vi "Update_Readback.vi"(8 "error in (no error)":errorcluster, 9 "Value":u32, 10 "PV URL":string, 11 "CS++IEFWerner in":refnum<class "CS++IEFWerner.lvclass">) -> (0 "error out":errorcluster, 3 "CS++IEFWerner out":refnum<class "CS++IEFWerner.lvclass">)   [LabVIEW 2015, in "CS++IEFWerner.lvlib" / "CS++IEFWerner.lvclass"]
doc: "This VI gets the infos from the Status SV of the IEF motor controller, makes some calculations and updates the important SVs."
uses:
  CS++IEFWerner.lvclass
  CS++IEFWerner.lvclass/CS++IEFWerner.ctl
  CSPP_Core/Classes/CS++ProcessVariables/ProcessVariable/PV.lvclass
  CSPP_Core/Classes/CS++ProcessVariables/ProcessVariable/PV.lvclass/PV.ctl
  CSPP_Core/Classes/CS++ProcessVariables/ProcessVariable/Write Data.vi
  CSPP_Core/Classes/CS++ProcessVariables/ProcessVariable/Write Timestamp.vi
  CSPP_Core/Classes/CS++ProcessVariables/PVConnection/PVConnection.lvclass
  CSPP_DeviceBase/CS++Motor/CS++Motor.lvclass
  instr.lib/IEF-pac/IEF Werner.lvlib
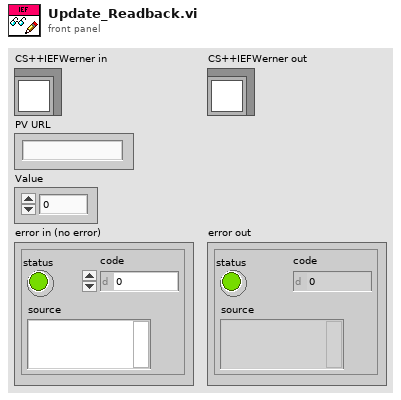
[diagram p1: front panel]
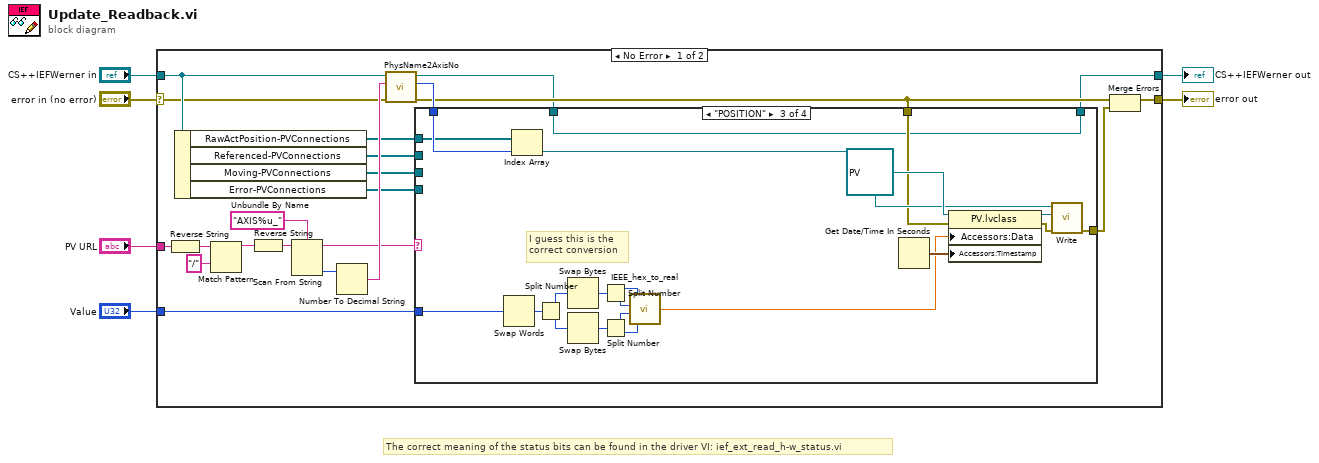
[diagram p0: block diagram]
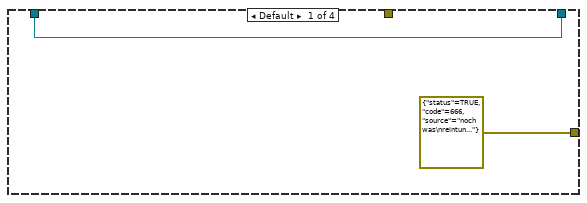
[diagram p2: hidden frame]
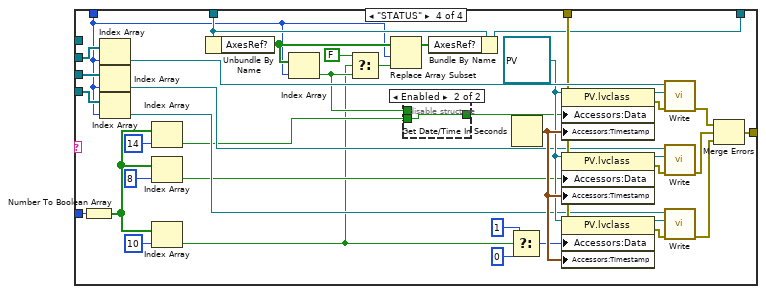
[diagram p4: hidden frame]
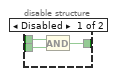
[diagram p5: hidden frame]
diagram:
  # "The correct meaning of the status bits can be found in the driver VI: ief_ext_read_h-w_status.vi"
  n1 = case shown="No Error" "error in (no error)" {
    selector: "error in (no error)" -> [w19 w97]
    tunnel: [w10 w97] -> w5
    tunnel: [w7 w96] -> w3
    tunnel: "CS++IEFWerner in" -> [w22 w96]
    tunnel: "PV URL" -> [w28 _]
    tunnel: "Value" -> [w12 _]
    frame No Error {
      n2 = Reverse String(1:w28) -> (0:w27:string)
      n3 = Unbundle By Name(w22) -> ("RawActPosition-PVConnections"=w16:refnum<class "PVConnection.lvclass">[], "Referenced-PVConnections"=w15:refnum<class "PVConnection.lvclass">[], "Moving-PVConnections"=w14:refnum<class "PVConnection.lvclass">[], "Error-PVConnections"=w13:refnum<class "PVConnection.lvclass">[])
      n4 = Match Pattern(string=w27, regular expression="/") -> (before substring=w26:string)  [unwired: 1 in, 3 out]
      n5 = Reverse String(1:w26) -> (0:w24:string)
      n6 = Scan From String(format string="AXIS%u_", input string=w24) -> (remaining string=w18:string, output 1=w21:u32)  [unwired: 3 in, 2 out]
      n7 = Number To Decimal String(number=w21) -> (decimal integer string=w20:string)  [unwired: 1 in]
      n8 = call "PhysName2AxisNo.vi"("error in (no error)"=w19, "PhysicalChannelName"=w20, "CS++Motor in"=w22) -> ("error out"=w11:errorcluster, "AxisNumber"=w17:u8, "CS++Motor out"=w8:refnum<class "CS++IEFWerner.lvclass">)  [unwired: 6 in]
      n9 = case shown="\"POSITION\"" w18 {
        tunnel: w17 -> [_ _ w48 w65]
        tunnel: w16 -> [_ _ w47 _]
        tunnel: w15 -> [_ _ _ w88]
        tunnel: w14 -> [_ _ _ w87]
        tunnel: w13 -> [_ _ _ w86]
        tunnel: w11 -> [_ _ w45 w79]
        tunnel: w12 -> [_ _ w34 w58]
        tunnel: [errorcluster {"status"=TRUE, "code"=666, "source"="noch was\nreintun..."} ("error out") _ w44 w72] -> w9
        tunnel: w8 -> [w29 w31 w32 w69]
        tunnel: [w29 w31 w32 w68] -> w7
        frame Default {
        }
        frame "\u0000" {
        }
        frame "POSITION" {
          # "I guess this is the\ncorrect conversion"
          n10 = Swap Words(1:w34) -> (0:w37:u32)
          n11 = Index Array(array=w47, index=w48) -> (element=w46:refnum<class "PVConnection.lvclass">)
          n12 = Split Number(x=w37) -> (hi(x)=w43:u16, lo(x)=w42:u16)
          n13 = Swap Bytes(anything=w43) -> (byte swapped=w36:u16)
          n14 = Swap Bytes(anything=w42) -> (byte swapped=w35:u16)
          n15 = Split Number(x=w36) -> (hi(x)=w38:u8, lo(x)=w40:u8)
          n16 = Split Number(x=w35) -> (hi(x)=w41:u8, lo(x)=w39:u8)
          n17 = call "IEEE_hex_to_real.vi"("number 4"=w39, "number 3"=w41, "number 2"=w40, "number"=w38) -> ("number 5"=w33:sgl)
          n18 = Get Date/Time In Seconds() -> (seconds since 1Jan1904=w50:timestamp)
          n19 = property class="PV.lvclass"(reference=refnum<class "PV.lvclass"> refnum ("PV"), error in=w45, "Accessors:Data"=w33, "Accessors:Timestamp"=w50) -> (reference out=w52:refnum<class "PV.lvclass">, error out=w51:errorcluster)
          n20 = call "Write.vi"("error in (no error)"=w51, "PV"=w52, "PVConnection in"=w46) -> ("error out"=w44:errorcluster)  [unwired: 7 in, 1 out]
        }
        frame "STATUS" {
          w80 = refnum<class "PV.lvclass"> refnum ("PV")
          n21 = Number To Boolean Array(number=w58) -> (Boolean array=w55:bool[])
          n22 = Index Array(array=w88, index=w65) -> (element=w89:refnum<class "PVConnection.lvclass">)
          n23 = Index Array(array=w87, index=w65) -> (element=w78:refnum<class "PVConnection.lvclass">)
          n24 = Index Array(array=w86, index=w65) -> (element=w77:refnum<class "PVConnection.lvclass">)
          n25 = Index Array(array=w55, index=14) -> (element=w54:bool)
          n26 = Index Array(array=w55, index=8) -> (element=w57:bool)
          n27 = Index Array(array=w55, index=10) -> (element=w53:bool)
          n28 = Unbundle By Name(w69) -> ("AxesRef?"=w67:bool[])
          n29 = Index Array(array=w67, index=w65) -> (element=w62:bool)
          n30 = Select(t=FALSE, s=w53, f=w62) -> (s? t:f=w64:bool)
          n31 = Replace Array Subset(array=w67, new element=w64, index=w65) -> (w66:bool[])
          n32 = disable-structure shown="Enabled" {
            disable-tunnel: w62 -> [w94 _]
            disable-tunnel: [w93 w95] -> w61
            disable-tunnel: w54 -> [w92 w95]
            frame Disabled {
              n33 = And(x=w94, y=w92) -> (x .and. y?=w93:bool)
            }
            frame Enabled {
            }
          }
          n34 = Bundle By Name(cluster=w69, "AxesRef?"=w66) -> (w68:refnum<class "CS++IEFWerner.lvclass">)
          n35 = Select(t=i8 1, s=w53, f=i8 0) -> (s? t:f=w74:i8)
          n36 = Get Date/Time In Seconds() -> (seconds since 1Jan1904=w81:timestamp)
          n37 = property class="PV.lvclass"(reference=w80, error in=w79, "Accessors:Data"=w61, "Accessors:Timestamp"=w81) -> (reference out=w91:refnum<class "PV.lvclass">, error out=w90:errorcluster)
          n38 = property class="PV.lvclass"(reference=w80, error in=w79, "Accessors:Data"=w57, "Accessors:Timestamp"=w81) -> (reference out=w84:refnum<class "PV.lvclass">, error out=w85:errorcluster)
          n39 = property class="PV.lvclass"(reference=w80, error in=w79, "Accessors:Data"=w74, "Accessors:Timestamp"=w81) -> (reference out=w83:refnum<class "PV.lvclass">, error out=w82:errorcluster)
          n40 = call "Write.vi"("error in (no error)"=w90, "PV"=w91, "PVConnection in"=w89) -> ("error out"=w73:errorcluster)  [unwired: 7 in, 1 out]
          n41 = call "Write.vi"("error in (no error)"=w85, "PV"=w84, "PVConnection in"=w78) -> ("error out"=w71:errorcluster)  [unwired: 7 in, 1 out]
          n42 = call "Write.vi"("error in (no error)"=w82, "PV"=w83, "PVConnection in"=w77) -> ("error out"=w70:errorcluster)  [unwired: 7 in, 1 out]
          n43 = Merge Errors(w73, w71, w70) -> (w72:errorcluster)
        }
      }
      n44 = Merge Errors(w11, w9) -> (w10:errorcluster)
    }
    frame Error {
    }
  }
  "error out" <- w5
  "CS++IEFWerner out" <- w3
